vi "RightClick.vi"(7 "isDisabled?":bool, 8 "error in (no error)":errorcluster, 9 "Table CtlRef In":refnum<vi>, 10 "Cell Position":T1, 11 "Column in":refnum<class "Column.lvclass">) -> (0 "error out":errorcluster, 1 "Table CtlRef Out":refnum<vi>, 2 "Discard?":bool, 3 "Column out":refnum<class "Column.lvclass">)   [LabVIEW 2013, in "Column.lvclass"]
uses:
  Column.lvclass
  <vilib>/Utility/miscctls.llb/LVRowAndColumnTypeDef.ctl
panel:
  # "Placeholder for now!\nWe want to implement custom contextual \nmenu upon right-click as generic behavior."
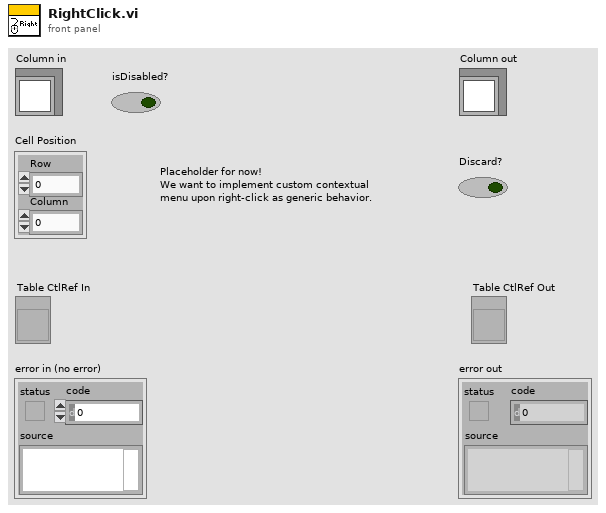
[diagram p1: front panel]
types:
  T1 = typedef "LVRowAndColumnTypeDef.ctl" = cluster{"Row":i32, "Column":i32}
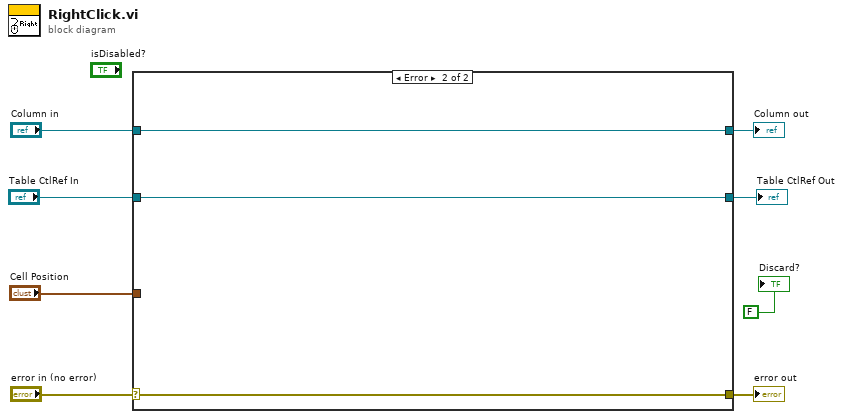
[diagram p0: block diagram]
diagram:
  n1 = case shown="Error" "error in (no error)" {
    selector: "error in (no error)" -> [w10 w14]
    tunnel: [w10 w14] -> w7
    tunnel: [w11 w13] -> w5
    tunnel: "Column in" -> [w11 w13]
    tunnel: "Table CtlRef In" -> [w9 w12]
    tunnel: [w9 w12] -> w3
    tunnel: "Cell Position" -> [_ _]
    frame No Error {
      # "By default, let LV handle.\n\nAdd more specific code for child classes."
      # "Wire the error cluster across even in the \"No Error\"\ncase so that warnings get propagated."
    }
    frame Error {
    }
  }
  "error out" <- w7
  "Column out" <- w5
  "Table CtlRef Out" <- w3
  "Discard?" <- FALSE ("Discard?")
